vi "Flyweight_Main.vi"() -> ()   [LabVIEW 2012]
uses:
  Row_class/Row.lvclass
  Character_class/Character.lvclass
  Glyph_class/Position.ctl
  <vilib>/event_ctls.llb/lveventtype.ctl
  GlyphFactory_class/GlyphFactory.lvclass
  Glyph_class/Glyph.lvclass
panel:
  in  "Font":enum16{"Arial", "Times New Roman"}(ring)
  in  "Font":T1={"Font Name:"="Arial", "Size"=24, "Strikeout?"=FALSE, "Italic?"=FALSE, "Underline?"=FALSE, "Outline?"=FALSE, "Shadow?"=FALSE, "Bold?"=FALSE}
  in  "Text Color":u32(colorbox)
  in  "ErrorIn":errorcluster
  out "ErrorOut":errorcluster
  in  "Text":picture
  # "*Show Debugger\n*Show Debug Control"
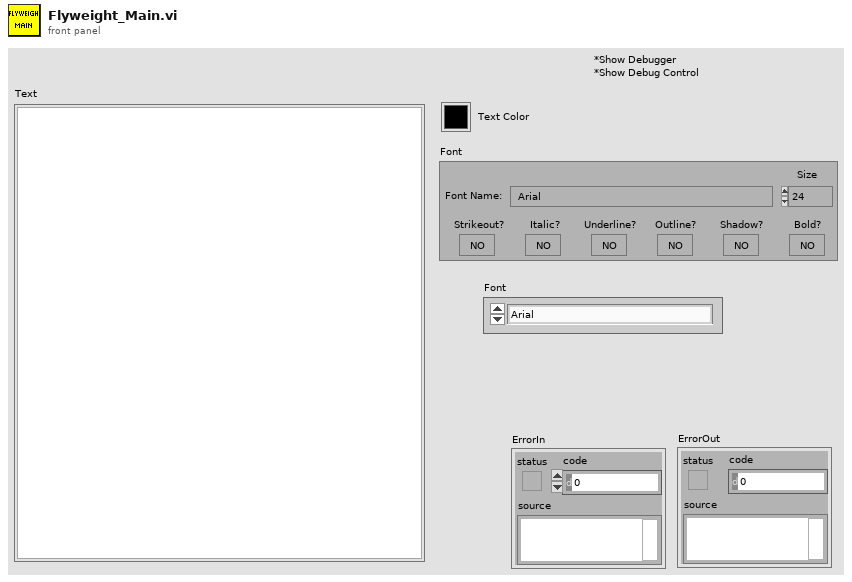
[diagram p1: front panel]
types:
  T1 = cluster{"Font Name:":string, "Size":i16, "Strikeout?":bool, "Italic?":bool, "Underline?":bool, "Outline?":bool, "Shadow?":bool, "Bold?":bool}
  T2 = cluster{"Text":string, "Cancelled":bool, "Rows":refnum<class "Row.lvclass">[], "LastPicture":picture, "Cursor":bool, "Focus":bool}
  T3 = typedef "Glyph.lvclass/Position.ctl" = cluster{"X":i32, "Y":i32}
  T4 = typedef "lveventtype.ctl" = enum32{"Null", "Timeout", "Annotation Menu Selection", "Annotation Menu Selection?", "App Instance Close", "App Instance Close?", "Autoscale Range Change", "Cell Edit", "Cell Edit?", "Cursor Grab", "Cursor Grab?", "Cursor Menu Selection", "Cursor Menu Selection?", "Cursor Move", "Cursor Release", "Data Change", "Direction Change", "Display State Change", "Drag Ended", "Drag Enter", "Drag Leave", "Drag Over", "Drag Source Update", "Drag Starting", "Drag Starting?", "Drop", "Exec State Change", "Key Down", "Key Down?", "Key Repeat", "Key Repeat?", "Key Up", "Listbox Double Click", "Menu Activation?", "Menu Selection (App)", "Menu Selection? (App)", "Menu Selection (User)", "Mouse Down", "Mouse Down?", "Mouse Enter", "Mouse Leave", "Mouse Move", "Mouse Up", "NI Security User Change (App)", "Pane Size", "Panel Close", "Panel Close?", "Panel Resize", "Plot Attribute Change", "Scale Range Change", "Shortcut Menu Activation?", "Shortcut Menu Selection (App)", "Shortcut Menu Selection? (App)", "Shortcut Menu Selection (User)", "Tree Double Click", "Tree Drag", "Tree Drag?", "Tree Drop", "Tree Drop?", "Tree Item Close", "Tree Item Close?", "Tree Item Open", "Tree Item Open?", "Value Change"}
  T5 = cluster{"Width":u16, "Style":enum32{"Solid", "Dash", "Dot", "DashDot", "DashDotDot"}}
  T6 = typedef "eventvkey.ctl" = enum16{"ASCII", "Enter", "Return", "Shift", "Ctrl", "Alt", "Cmd", "Opt", "Caps", "NumLock", "Clear", "Break", "Up", "Down", "Left", "Right", "Insert", "Delete", "Home", "End", "PageUp", "PageDown", "Escape", "Help", "Pause", "ScrollLock", "F1", "F2", "F3", "F4", "F5", "F6", "F7", "F8", "F9", "F10", "F11", "F12", "F13", "F14", "F15", "F16", "F17", "F18", "F19", "F20", "F21", "F22", "F23", "F24", "Play", "VolumeUp", "VolumeDown", "Mute", "Two Byte Char"}
  T7 = typedef "Glyph.lvclass/Dimensions.ctl" = cluster{"Width":i32, "Height":i32}
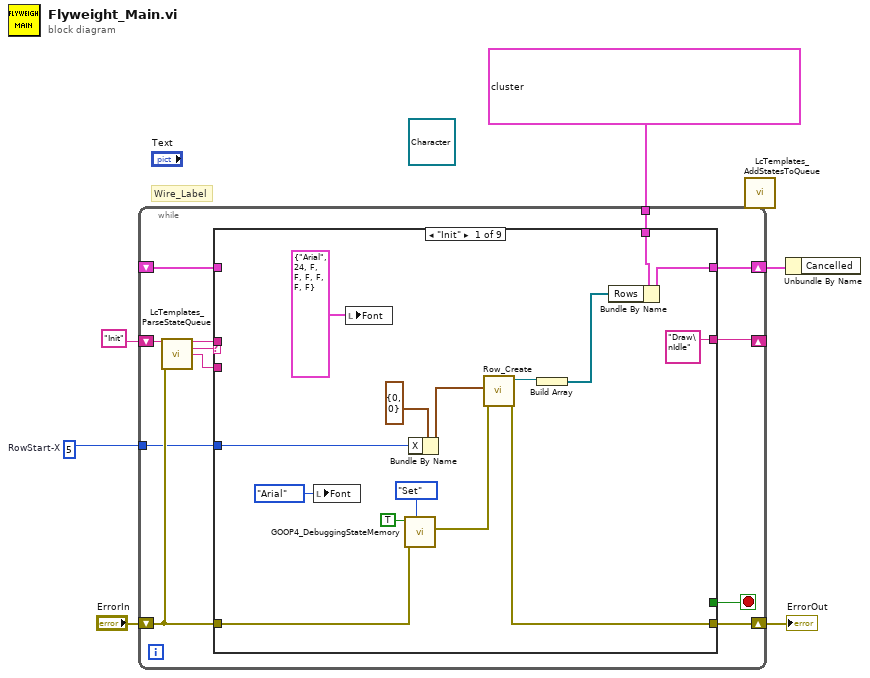
[diagram p0: block diagram]
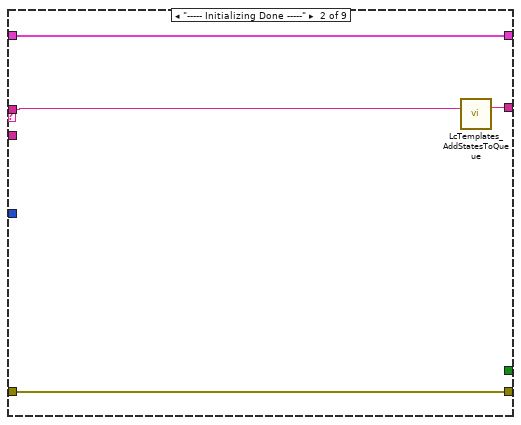
[diagram p2: hidden frame]
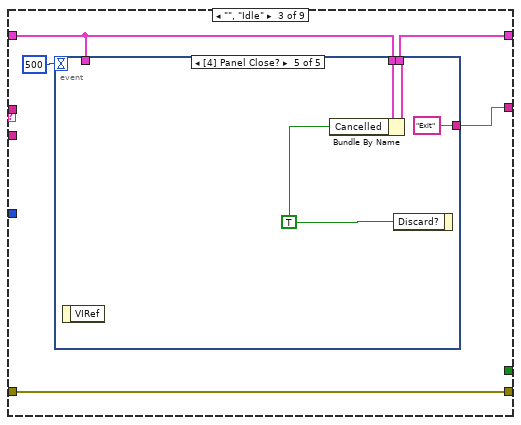
[diagram p3: hidden frame]
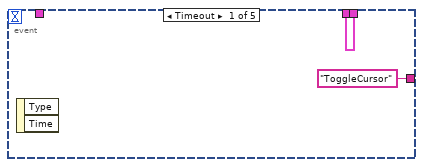
[diagram p4: hidden frame]
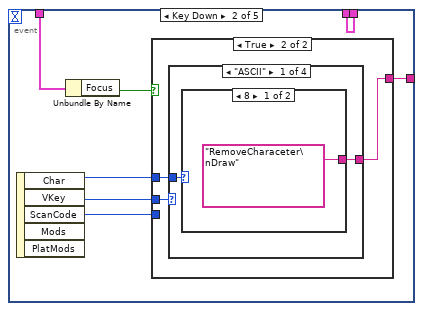
[diagram p5: hidden frame]
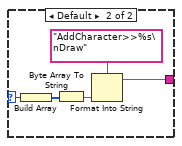
[diagram p7: hidden frame]
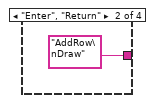
[diagram p8: hidden frame]
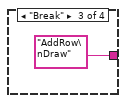
[diagram p9: hidden frame]
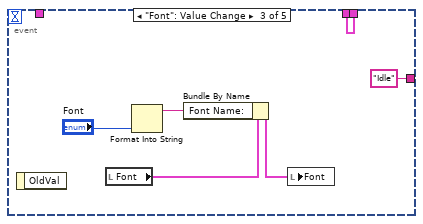
[diagram p11: hidden frame]
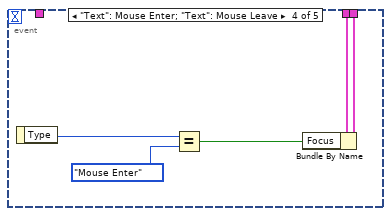
[diagram p12: hidden frame]
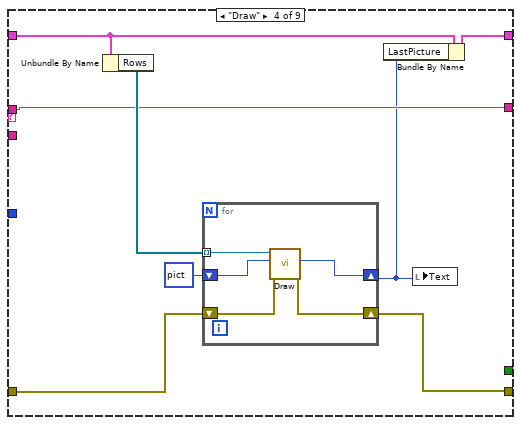
[diagram p13: hidden frame]
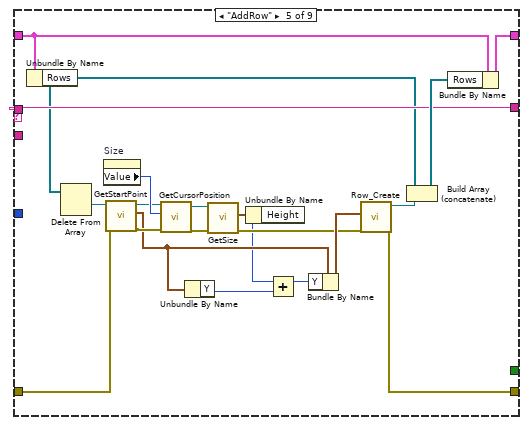
[diagram p14: hidden frame]
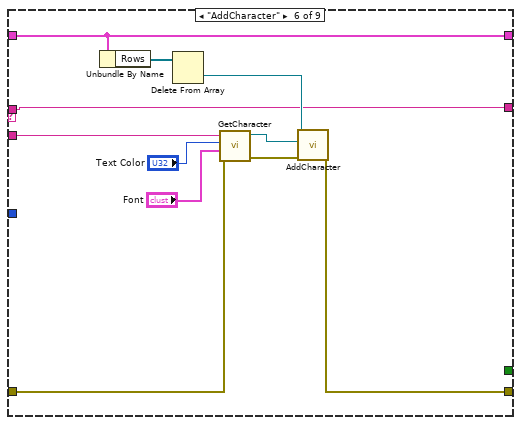
[diagram p15: hidden frame]
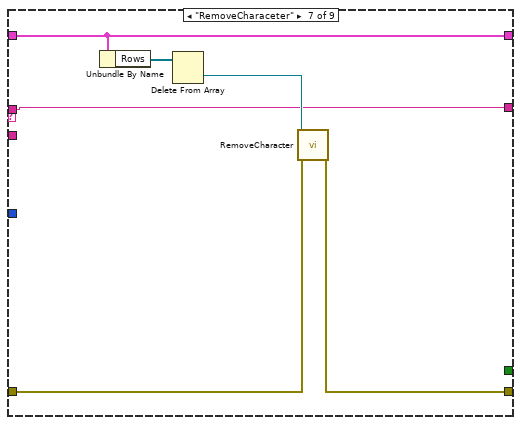
[diagram p16: hidden frame]
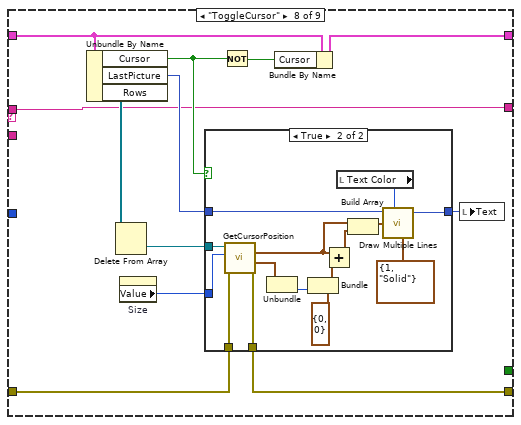
[diagram p17: hidden frame]
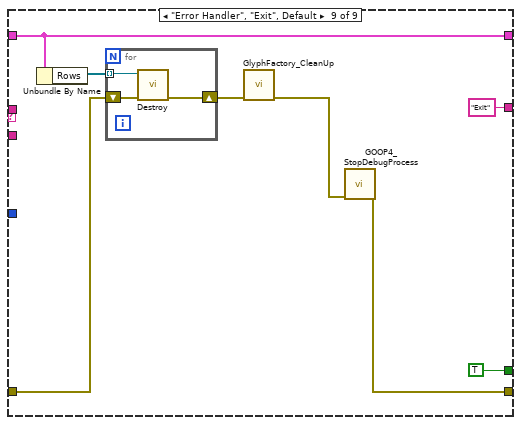
[diagram p19: hidden frame]
diagram:
  w1 = 5  # RowStart-X
  (unwired) refnum<class "Character.lvclass"> refnum ("Character")
  # "Wire_Label"
  n1 = while {
    shift-right: [w18] -> w5
    shift-left: "ErrorIn" -> [w9]
    shift-right: [w10] -> _
    shift-left: "Init" -> [w15]
    shift-right: [w17] -> w4
    shift-left: _ -> [w16]
    tunnel: T2 {"Text"="", "Cancelled"=FALSE, "Rows"=[], "LastPicture"=bytes[0], "Cursor"=FALSE, "Focus"=FALSE} -> [w12]
    tunnel: w1 -> [w7]
    stop <- w8 stop-if-true
    n2 = call <userlib>:"LcTemplates_ParseStateQueue.vi"("State Queue"=w15, "Error In (no error)"=w9) -> ("Remaining States"=w11:string, "Current State"=w14:string, "Arguments"=w13:string)  [unwired: 11 out]
    n3 = case shown="\"Init\"" w14 {
      tunnel: w9 -> [w20 w34 w41 w85 w105 w121 w125 w134 w161]
      tunnel: [w28 w34 w41 w84 w98 w116 w128 w133 w160] -> w18
      tunnel: [w33 w35 w42 w81 w110 w114 w126 w140 w165] -> w17
      tunnel: w16 -> [_ w35 w38 w82 w112 w114 w126 w142 w165]
      tunnel: w13 -> [_ _ _ _ _ w124 _ _ _]
      tunnel: w12 -> [w32 _ _ _ _ _ _ _ _]
      tunnel: w11 -> [_ w36 _ w83 w109 w115 w127 w132 _]
      tunnel: ["Draw\nIdle" w37 w40 w83 w109 w115 w127 w132 "Exit"] -> w10
      tunnel: [_ _ _ _ _ _ _ _ TRUE] -> w8
      tunnel: w7 -> [w25 _ _ _ _ _ _ _ _]
      frame "Init" {
        n4 = local write "Font"(enum16{"Arial", "Times New Roman"}."Arial" ("Font")) -> ()
        n5 = local write "Font"(T1 {"Font Name:"="Arial", "Size"=24, "Strikeout?"=FALSE, "Italic?"=FALSE, "Underline?"=FALSE, "Outline?"=FALSE, "Shadow?"=FALSE, "Bold?"=FALSE} ("Font")) -> ()
        n6 = call <vilib>:"GOOP4_DebuggingStateMemory.vi"("Action(Read)"=enum16{"Read", "Set"}."Set", "error in (no error)"=w20, "DebuggingStateIn"=TRUE) -> ("error out"=w19:errorcluster)  [unwired: 7 in, 1 out]
        n7 = Bundle By Name(cluster=T3 {"X"=0, "Y"=0} ("StartPoint"), "X"=w25) -> (w23:T3)
        n8 = call "Row_Create.vi"("error in (no error)"=w19, "StartPoint"=w23) -> ("error out"=w28:errorcluster, "reference out"=w27:refnum<class "Row.lvclass">)  [unwired: 8 in]
        n9 = Build Array(w27) -> (w26:refnum<class "Row.lvclass">[])
        n10 = Bundle By Name(cluster=w32, "Rows"=w26) -> (w33:T2)
      }
      frame "----- Initializing Done -----" {
        n11 = call <userlib>:"LcTemplates_AddStatesToQueue.vi"("State(s) in (\"\")"=w36) -> ("States Out"=w37:string)  [unwired: 2 in, 12 out]
      }
      frame "", "Idle" {
        n12 = event shown="[4] Panel Close?" {
          selector: _ -> [_ _ _ _ _]
          dyn-events: _ -> [_ _ _ _ _]
          timeout: 500 -> [_ _ _ _ _]
          tunnel: w38 -> [w44 w45 w65 w75 w78]
          tunnel: [w44 w45 w65 w74 w77] -> w42
          tunnel: ["ToggleCursor" w50 "Idle" _ "Exit"] -> w40
          tunnel: w38 -> [_ w48 _ _ _]
          event Timeout {
            n13 = event-data() -> ()  [unwired: 3 out]
          }
          event Key Down {
            n14 = event-data() -> ("Char"=w49:i16, "VKey"=w51:T6, "ScanCode"=w46:i16)  [unwired: 3 out]
            n15 = Unbundle By Name(w48) -> ("Focus"=w47:bool)
            n16 = case shown="True" w47 {
              tunnel: w51 -> [_ w54]
              tunnel: [_ w53] -> w50
              tunnel: w49 -> [_ w52]
              tunnel: w46 -> [_ _]
              frame False {
              }
              frame True {
                n17 = case shown="\"ASCII\"" w54 {
                  tunnel: [w56 "AddRow\nDraw" "AddRow\nDraw" _] -> w53
                  tunnel: w52 -> [w55 _ _ _]
                  frame "ASCII" {
                    n18 = case shown="8" w55 {
                      selector: w55 -> [_ w58]
                      tunnel: ["RemoveCharaceter\nDraw" w61] -> w56
                      frame 8 {
                      }
                      frame Default {
                        n19 = Build Array(w58) -> (w59:i16[])
                        n20 = Byte Array To String(unsigned byte array=w59) -> (string=w60:string)
                        n21 = Format Into String(format string="AddCharacter>>%s\nDraw", w60) -> (resulting string=w61:string)  [unwired: 2 in, 1 out]
                      }
                    }
                  }
                  frame "Enter", "Return" {
                  }
                  frame "Break" {
                  }
                  frame Default {
                  }
                }
              }
            }
          }
          event "Font": Value Change {
            n22 = event-data() -> ()  [unwired: 2 out]
            n23 = local read "Font"() -> (w69:T1)
            n24 = Format Into String("Font") -> (resulting string=w67:string)  [unwired: 3 in, 1 out]
            n25 = Bundle By Name(cluster=w69, "Font Name:"=w67) -> (w68:T1)
            n26 = local write "Font"(w68) -> ()
          }
          event "Text": Mouse Enter; "Text": Mouse Leave {
            n27 = event-data() -> ("Type"=w73:T4)  [unwired: 1 out]
            n28 = Equal?(x=w73, y=lveventtype."Mouse Enter") -> (x = y?=w71:bool)
            n29 = Bundle By Name(cluster=w75, "Focus"=w71) -> (w74:T2)
          }
          event Panel Close? {
            w76 = TRUE ("Discard?")
            n30 = event-data() -> ()  [unwired: 2 out]
            n31 = Bundle By Name(cluster=w78, "Cancelled"=w76) -> (w77:T2)
            n32 = event-data("Discard?"=w76) -> ()  [unwired: 1 in, 1 out]
          }
        }
      }
      frame "Draw" {
        n33 = Unbundle By Name(w82) -> ("Rows"=w87:refnum<class "Row.lvclass">[])
        n34 = for {
          tunnel: w87 -> [w92] mode=indexing
          shift-right: [w91] -> w80
          shift-left: picture data[5B] ("PictureOut") -> [w90]
          shift-right: [w88] -> w84
          shift-left: w85 -> [w89]
          n35 = call-dynamic "Draw.vi"("error in (no error)"=w89, "PictureIn"=w90, "reference in"=w92) -> ("error out"=w88:errorcluster, "PictureOut"=w91:picture)  [unwired: 5 in, 2 out]
        }
        n36 = Bundle By Name(cluster=w82, "LastPicture"=w80) -> (w81:T2)
        n37 = local write "Text"(w80) -> ()
      }
      frame "AddRow" {
        n38 = Unbundle By Name(w112) -> ("Rows"=w108:refnum<class "Row.lvclass">[])
        n39 = Delete From Array(array=w108) -> (deleted portion=w106:refnum<class "Row.lvclass">)  [unwired: 2 in, 1 out]
        n40 = property on="Size" class="DigNum (strict)"() -> ("Value"=w107:i16)  [unwired: 2 in, 2 out]
        n41 = call-dynamic "GetStartPoint.vi"("error in (no error)"=w105, "reference in"=w106) -> ("error out"=w103:errorcluster, "StartPoint"=w96:T3, "reference in"=w104:refnum<class "Row.lvclass">)  [unwired: 7 in]
        n42 = call-dynamic "GetCursorPosition.vi"("error in (no error)"=w103, "DefaultHeight"=w107, "reference in"=w104) -> ("error out"=w101:errorcluster, "reference in"=w100:refnum<class "Row.lvclass">)  [unwired: 5 in, 2 out]
        n43 = Unbundle By Name(w96) -> ("Y"=w95:i32)
        n44 = call-dynamic "GetSize.vi"("error in (no error)"=w101, "reference in"=w100) -> ("error out"=w99:errorcluster, "Dimensions"=w97:T7)  [unwired: 7 in, 1 out]
        n45 = Unbundle By Name(w97) -> ("Height"=w94:i32)
        n46 = Add(x=w94, y=w95) -> (x+y=w93:i32)
        n47 = Bundle By Name(cluster=w96, "Y"=w93) -> (w102:T3)
        n48 = call "Row_Create.vi"("error in (no error)"=w99, "StartPoint"=w102) -> ("error out"=w98:errorcluster, "reference out"=w113:refnum<class "Row.lvclass">)  [unwired: 8 in]
        n49 = Build Array (concatenate)(w108, w113) -> (w111:refnum<class "Row.lvclass">[])
        n50 = Bundle By Name(cluster=w112, "Rows"=w111) -> (w110:T2)
      }
      frame "AddCharacter" {
        n51 = Unbundle By Name(w114) -> ("Rows"=w120:refnum<class "Row.lvclass">[])
        n52 = Delete From Array(array=w120) -> (deleted portion=w119:refnum<class "Row.lvclass">)  [unwired: 2 in, 1 out]
        n53 = call "GetCharacter.vi"("error in (no error)"=w121, "Font"="Font", "Text Color"="Text Color", "Char"=w124) -> ("error out"=w117:errorcluster, "Character"=w118:refnum<class "Character.lvclass">)  [unwired: 6 in]
        n54 = call-dynamic "AddCharacter.vi"("error in (no error)"=w117, "Character"=w118, "reference in"=w119) -> ("error out"=w116:errorcluster)  [unwired: 7 in, 1 out]
      }
      frame "RemoveCharaceter" {
        n55 = Unbundle By Name(w126) -> ("Rows"=w130:refnum<class "Row.lvclass">[])
        n56 = Delete From Array(array=w130) -> (deleted portion=w129:refnum<class "Row.lvclass">)  [unwired: 2 in, 1 out]
        n57 = call-dynamic "RemoveCharacter.vi"("error in (no error)"=w125, "reference in"=w129) -> ("error out"=w128:errorcluster)  [unwired: 8 in, 1 out]
      }
      frame "ToggleCursor" {
        n58 = Unbundle By Name(w142) -> ("Cursor"=w139:bool, "LastPicture"=w138:picture, "Rows"=w136:refnum<class "Row.lvclass">[])
        n59 = Delete From Array(array=w136) -> (deleted portion=w135:refnum<class "Row.lvclass">)  [unwired: 2 in, 1 out]
        n60 = property on="Size" class="DigNum (strict)"() -> ("Value"=w131:i16)  [unwired: 2 in, 2 out]
        n61 = case shown="True" w139 {
          tunnel: w138 -> [w144 w158]
          tunnel: [w144 w157] -> w137
          tunnel: w135 -> [_ w159]
          tunnel: w134 -> [w143 w153]
          tunnel: [w143 w152] -> w133
          tunnel: w131 -> [_ w145]
          frame False {
          }
          frame True {
            n62 = call-dynamic "GetCursorPosition.vi"("error in (no error)"=w153, "DefaultHeight"=w145, "reference in"=w159) -> ("error out"=w152:errorcluster, "Dimensions"=w147:T7, "CursorStartPoint"=w151:T3)  [unwired: 5 in, 1 out]
            n63 = Unbundle(w147) -> ("Height"=w146:i32)  [unwired: 1 out]
            n64 = Bundle(cluster=T3 {"X"=0, "Y"=0} ("StartPoint"), "Y"=w146) -> (w148:T3)  [unwired: 1 in]
            n65 = Add(x=w151, y=w148) -> (x+y=w150:T3)
            n66 = local read "Text Color"() -> (w155:u32)
            n67 = Build Array(w151, w150) -> (w154:T3[])
            n68 = call <vilib>:"Draw Multiple Lines.vi"("picture"=w158, "line endpoints"=w154, "color(black)"=w155, "pen"=T5 {"Width"=1, "Style"=enum."Solid"}) -> ("new picture"=w157:picture)  [unwired: 5 in]
          }
        }
        n69 = Not(x=w139) -> (.not. x?=w141:bool)
        n70 = Bundle By Name(cluster=w142, "Cursor"=w141) -> (w140:T2)
        n71 = local write "Text"(w137) -> ()
      }
      frame "Error Handler", "Exit", Default {
        n72 = Unbundle By Name(w165) -> ("Rows"=w164:refnum<class "Row.lvclass">[])
        n73 = for {
          tunnel: w164 -> [w170] mode=indexing
          shift-right: [w168] -> w163
          shift-left: w161 -> [w169]
          n74 = call-dynamic "Destroy.vi"("error in (no error)"=w169, "reference in"=w170) -> ("error out"=w168:errorcluster)  [unwired: 8 in, 1 out]
        }
        n75 = call "GlyphFactory_CleanUp.vi"("error in (no error)"=w163) -> ("error out"=w162:errorcluster)  [unwired: 10 in]
        n76 = call <vilib>:"GOOP4_StopDebugProcess.vi"("error in"=w162) -> ("error out"=w160:errorcluster)  [unwired: 10 in]
      }
    }
  }
  "ErrorOut" <- w5
  n77 = call <userlib>:"LcTemplates_AddStatesToQueue.vi"() -> ()  [unwired: 4 in, 12 out]
  n78 = Unbundle By Name(w4) -> ()  [unwired: 1 out]
